vi "CreateClonedHierarchyFromChildItem.vi"(8 "error in (no error)":errorcluster, 9 "ILabVIEWItem to clone":refnum<class "ILabVIEWItem.lvclass">, 10 "Root path":path, 11 "CDependencyList in":refnum<class "CDependencyList.lvclass">) -> (0 "error out":errorcluster, 1 "Hierarchy items":refnum<class "ILabVIEWItem.lvclass">[](array[class]), 3 "CDependencyList out":refnum<class "CDependencyList.lvclass">)   [LabVIEW 2020, in "DependencyInspection.lvlib" / "CDependencyList.lvclass"]
uses:
  CDependencyList.lvclass
  LabVIEWObjectFactory/LabVIEWObjectFactory.lvlib
  LabVIEWObjectInterfaces/ILabVIEWItem/ILabVIEWItem.lvclass
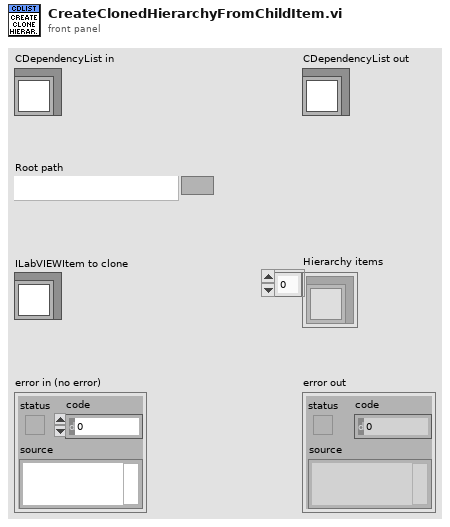
[diagram p1: front panel]
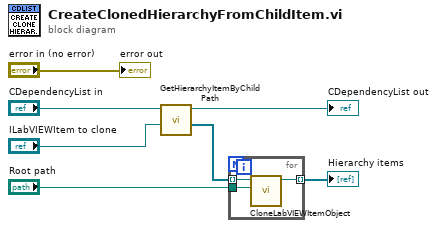
[diagram p0: block diagram]
diagram:
  n1 = call-dynamic "GetHierarchyItemByChildPath.vi"("Child ILabVIEWItem"="ILabVIEWItem to clone", "CDependencyList in"="CDependencyList in") -> ("Hierarchy items"=w3:refnum<class "ILabVIEWItem.lvclass">[], "CDependencyList out"=→"CDependencyList out":refnum<class "CDependencyList.lvclass">)  [unwired: 7 in, 1 out]
  n2 = for {
    tunnel: "Root path" -> [w10]
    tunnel: w3 -> [w9] mode=indexing
    tunnel: [w8] -> w1 mode=indexing
    n3 = call "CloneLabVIEWItemObject.vi"("Root path"=w10, "ILabVIEWItem in"=w9) -> ("Cloned ILabVIEWItem"=w8:refnum<class "ILabVIEWItem.lvclass">)  [unwired: 9 in]
  }
  "Hierarchy items" <- w1
  "error out" <- "error in (no error)"
